vi "VSG-AMPL_REF_SET.vi"(0 "VISA session":refnum<visa-resource-name>, 1 "Ampl Ref Set (0.00)":dbl format="%.2f", 2 "Ampl Ref (F:OFF)":bool, 3 "Ampl Offset (0.00)":dbl format="%.2f", 5 "Amplitude (-135.00)":dbl=-135.0 format="%.2f", 7 "Unit (0:dBm)":T1(ring), 9 "Atten Hold (F:OFF)":bool, 11 "error in (no error)":errorcluster {"code" format="%.0x"}) -> (4 "dup VISA session":refnum<visa-resource-name>, 15 "error out":errorcluster {"code" format="%.0x"})   [LabVIEW 2018]
doc: "This VI is used to set the modulation controls and the parameters associated with the signal generator's RF output amplitude."
panel:
  # "ON"
  # "OFF"
  # "ON"
  # "OFF"
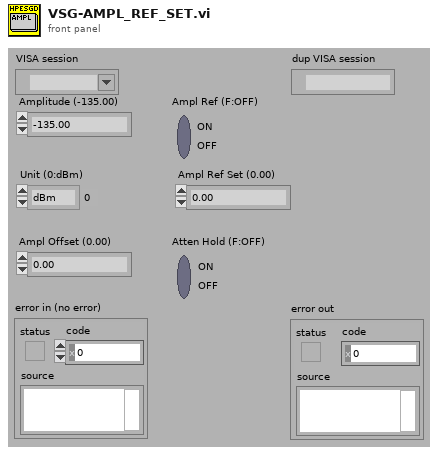
[diagram p1: front panel]
types:
  T1 = enum16{"dBm", "dBuV", "dBuVemf", "mV", "uV", "mVemf", "uVemf"}
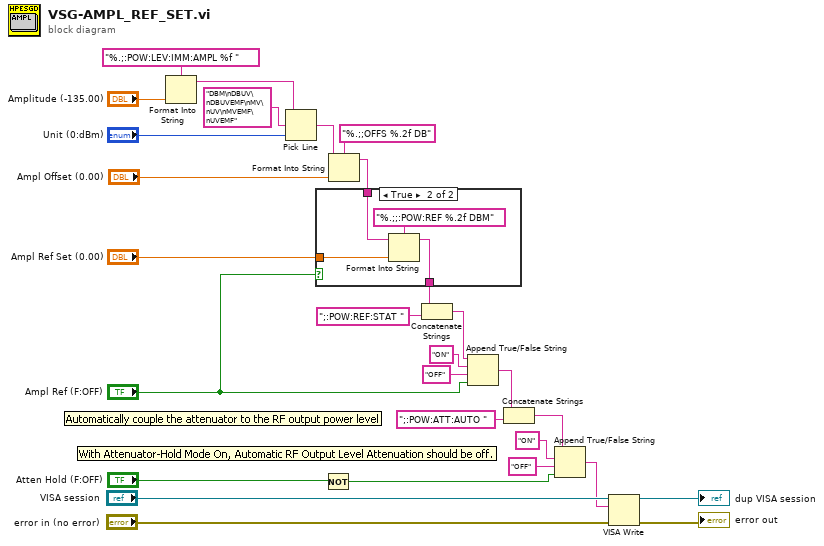
[diagram p0: block diagram]
diagram:
  n1 = Format Into String(format string="%.;:POW:LEV:IMM:AMPL %f ", "Amplitude (-135.00)") -> (resulting string=w21:string)  [unwired: 2 in, 1 out]
  n2 = Pick Line(string ("")=w21, multi-line string="DBM\nDBUV\nDBUVEMF\nMV\nUV\nMVEMF\nUVEMF", line index="Unit (0:dBm)") -> (output string=w24:string)
  n3 = Not(x="Atten Hold (F:OFF)") -> (.not. x?=w1:bool)
  n4 = Format Into String(format string="%.;;OFFS %.2f DB", initial string=w24, "Ampl Offset (0.00)") -> (resulting string=w7:string)  [unwired: 1 in, 1 out]
  n5 = case shown="True" "Ampl Ref (F:OFF)" {
    tunnel: w7 -> [w29 w32]
    tunnel: "Ampl Ref Set (0.00)" -> [_ w31]
    tunnel: [w29 w30] -> w5
    frame False {
    }
    frame True {
      n6 = Format Into String(format string="%.;;:POW:REF %.2f DBM", initial string=w32, w31) -> (resulting string=w30:string)  [unwired: 1 in, 1 out]
    }
  }
  n7 = Concatenate Strings(w5, ";:POW:REF:STAT ") -> (w3:string)
  n8 = Append True/False String(1:"Ampl Ref (F:OFF)", 2:"OFF" ("false string"), 3:"ON" ("true string"), 4:w3) -> (0:w14:string)
  n9 = Concatenate Strings(w14, ";:POW:ATT:AUTO ") -> (w13:string)
  n10 = Append True/False String(1:w1, 2:"OFF" ("false string"), 3:"ON" ("true string"), 4:w13) -> (0:w11:string)
  n11 = VISA Write(VISA resource name="VISA session", write buffer=w11, error in (no error)="error in (no error)") -> (VISA resource name out=→"dup VISA session":refnum<visa-resource-name>, error out=→"error out":errorcluster)  [unwired: 1 out]
